vi "Mechanism Log.vi"(10 "Co-Pilot Data in":T1, 11 "Byte Stream File in":refnum<file>) -> ()   [LabVIEW 2014]
uses:
  Co-Pilot_game_control.ctl
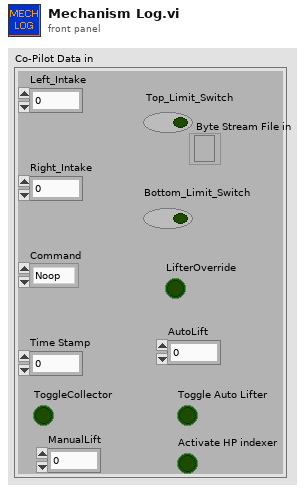
[diagram p1: front panel]
types:
  T1 = typedef "Co-Pilot_game_control.ctl" = cluster{"Left_Intake":dbl, "Right_Intake":dbl, "Time Stamp":u32, "Command":enum16{"Noop", "Flagged"}, "ToggleCollector":bool, "ManualLift":dbl, "Top_Limit_Switch":bool, "Bottom_Limit_Switch ":bool, "LifterOverride":bool, "AutoLift":i32, "Toggle Auto Lifter":bool, "Activate HP indexer":bool}
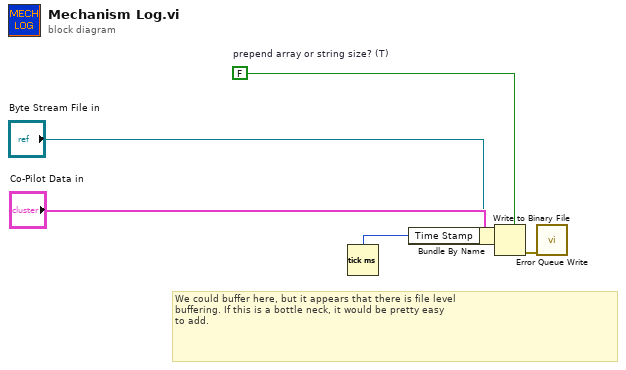
[diagram p0: block diagram]
diagram:
  w3 = FALSE  # prepend array or string size? (T)
  # "We could buffer here, but it appears that there is file level\nbuffering. If this is a bottle neck, it would be pretty easy\nto add."
  n1 = Tick Count (ms)() -> (millisecond timer value=w6:u32)
  n2 = Bundle By Name(cluster="Co-Pilot Data in", "Time Stamp"=w6) -> (w1:T1)
  n3 = Write to Binary File(file (use dialog)="Byte Stream File in", data=w1, 5:w3) -> (error out=w4:errorcluster)  [unwired: 3 in, 2 out]
  n4 = call "Error Queue Write.vi"("error in (no error)"=w4) -> ()  [unwired: 11 in]
